vi "GetValuesFromRefs.vi"(11 "ChangeonFly":T2) -> (3 "output cluster":T1)   [LabVIEW 2023]
uses:
  TypeDefs/ChangeOnFly.ctl
  User_Vi/Settings.vi
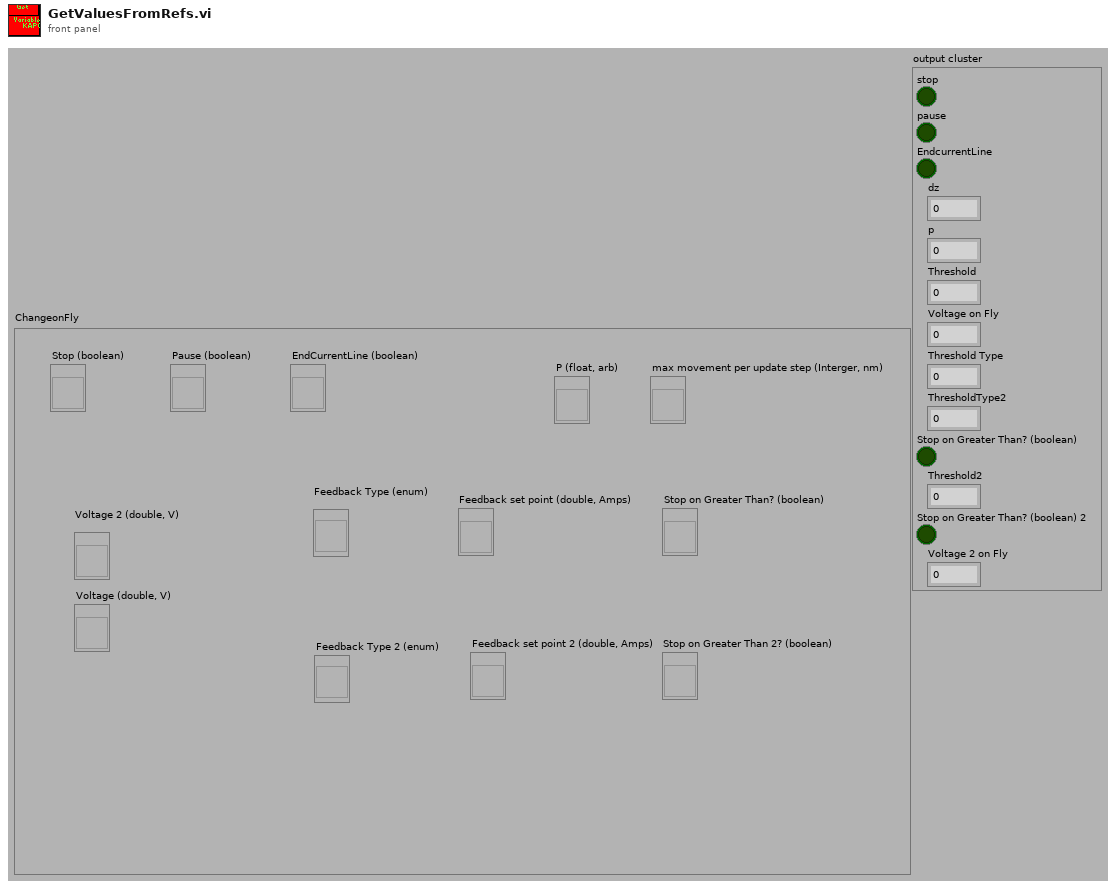
[diagram p1: front panel]
types:
  T1 = cluster{"stop":bool, "pause":bool, "EndcurrentLine":bool, "dz":i32, "p":fxp<+/-,32,1>, "Threshold":i64, "Voltage on Fly":i16, "Threshold Type":u8, "ThresholdType2":u8, "Stop on Greater Than? (boolean)":bool, "Threshold2":i64, "Stop on Greater Than? (boolean) 2":bool, "Voltage 2 on Fly":i16}
  T2 = typedef "ChangeOnFly.ctl" = cluster{"Stop (boolean)":refnum<vi>, "Pause (boolean)":refnum<vi>, "EndCurrentLine (boolean)":refnum<vi>, "max movement per update step (Interger, nm)":refnum<vi>, "P (float, arb)":refnum<vi>, "Feedback set point (double, Amps)":refnum<vi>, "Voltage (double, V)":refnum<vi>, "Feedback set point 2 (double, Amps)":refnum<vi>, "Stop on Greater Than 2? (boolean)":refnum<vi>, "Stop on Greater Than? (boolean)":refnum<vi>, "Voltage 2 (double, V)":refnum<vi>, "Feedback Type (enum)":refnum<vi>, "Feedback Type 2 (enum)":refnum<vi>}
  T3 = enum16{"AC Magnitude", "Current 1", "Current 2", "Phase"}
  T4 = typedef "Current Amplifier Settings.ctl" = dbl
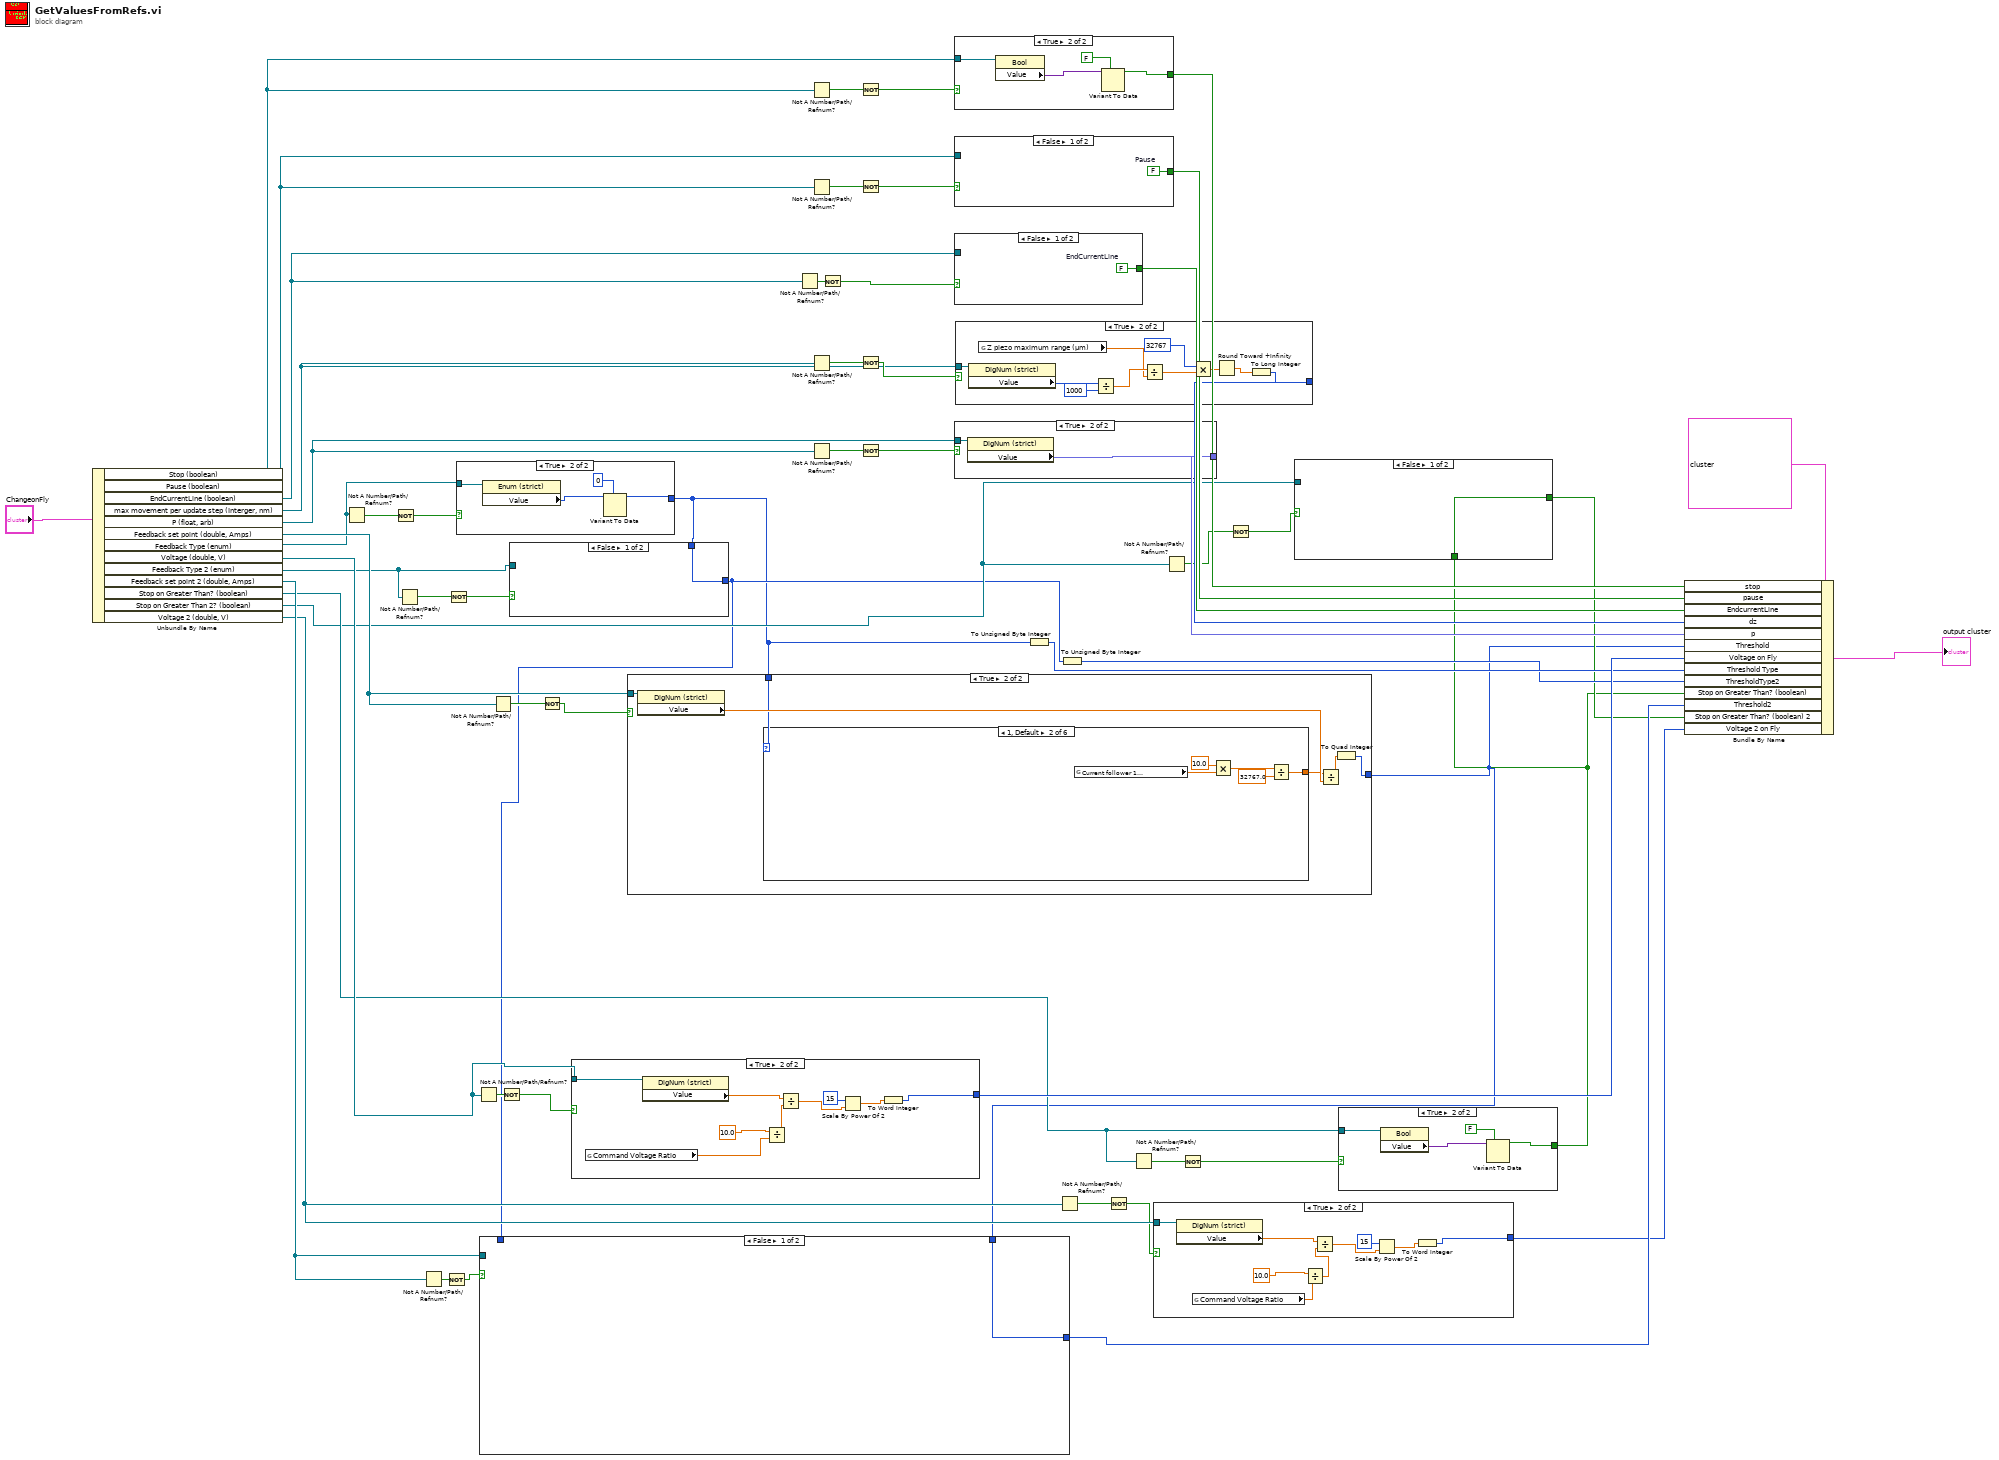
[diagram p0: block diagram]
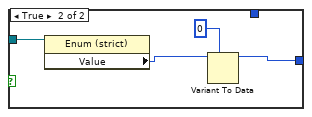
[diagram p2: hidden frame]
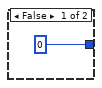
[diagram p3: hidden frame]
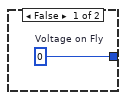
[diagram p4: hidden frame]
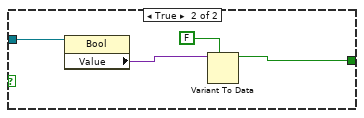
[diagram p5: hidden frame]
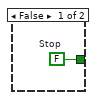
[diagram p6: hidden frame]
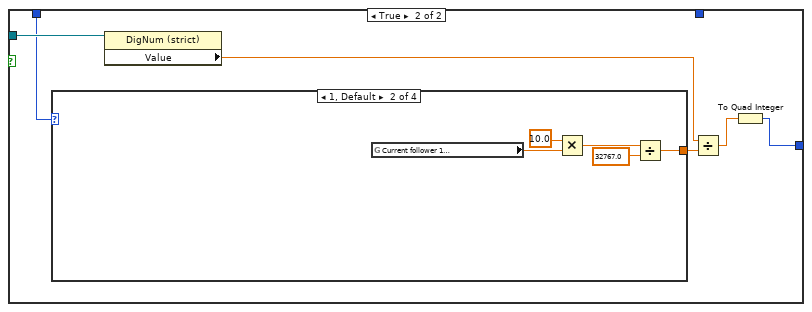
[diagram p7: hidden frame]
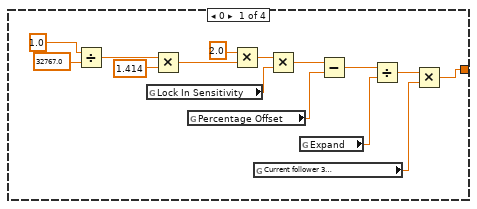
[diagram p8: hidden frame]
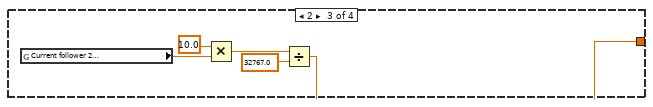
[diagram p9: hidden frame]
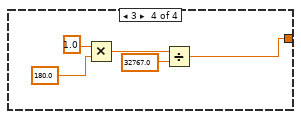
[diagram p10: hidden frame]
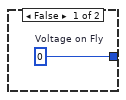
[diagram p11: hidden frame]
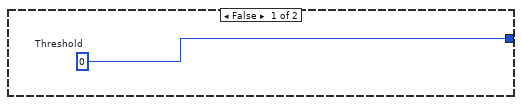
[diagram p12: hidden frame]
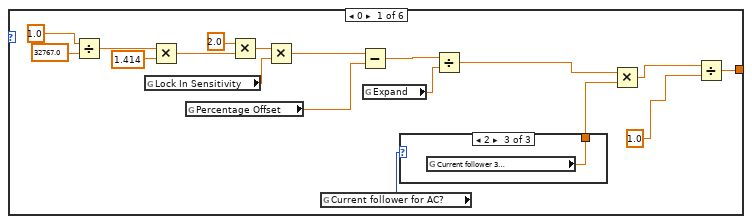
[diagram p13: hidden frame]
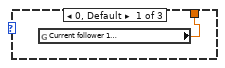
[diagram p14: hidden frame]
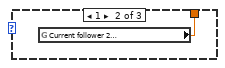
[diagram p15: hidden frame]
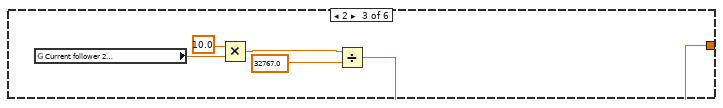
[diagram p16: hidden frame]
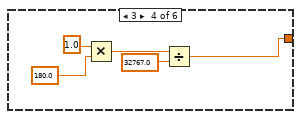
[diagram p17: hidden frame]
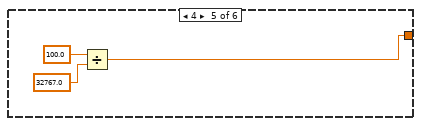
[diagram p18: hidden frame]
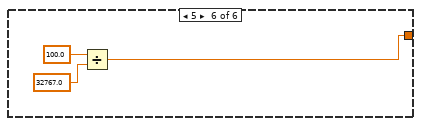
[diagram p19: hidden frame]
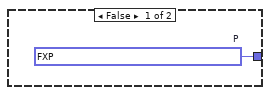
[diagram p20: hidden frame]
diagram:
  n1 = Unbundle By Name("ChangeonFly") -> ("Stop (boolean)"=w13:refnum<vi>, "Pause (boolean)"=w53:refnum<vi>, "EndCurrentLine (boolean)"=w50:refnum<vi>, "max movement per update step (Interger, nm)"=w47:refnum<vi>, "P (float, arb)"=w44:refnum<vi>, "Feedback set point (double, Amps)"=w36:refnum<vi>, "Feedback Type (enum)"=w10:refnum<vi>, "Voltage (double, V)"=w33:refnum<vi>, "Feedback Type 2 (enum)"=w9:refnum<vi>, "Feedback set point 2 (double, Amps)"=w25:refnum<vi>, "Stop on Greater Than? (boolean)"=w22:refnum<vi>, "Stop on Greater Than 2? (boolean)"=w19:refnum<vi>, "Voltage 2 (double, V)"=w15:refnum<vi>)
  n2 = Not A Number/Path/Refnum?(number/path/refnum=w10) -> (NaN/Path/Refnum?=w12:bool)
  n3 = Not(x=w12) -> (.not. x?=w11:bool)
  n4 = Not A Number/Path/Refnum?(number/path/refnum=w9) -> (NaN/Path/Refnum?=w8:bool)
  n5 = Not A Number/Path/Refnum?(number/path/refnum=w25) -> (NaN/Path/Refnum?=w30:bool)
  n6 = Not(x=w30) -> (.not. x?=w29:bool)
  n7 = Not(x=w8) -> (.not. x?=w7:bool)
  n8 = case shown="True" w11 {
    tunnel: w10 -> [_ w61]
    tunnel: [0 ("y") w59] -> w5
    frame False {
    }
    frame True {
      n9 = property on="Property Node" class="Enum (strict)"(reference=w61) -> ("Value"=w62:T3)  [unwired: 1 in, 2 out]
      n10 = Variant To Data(type=0 ("y"), Variant=w62) -> (data=w59:i32)  [unwired: 1 in, 1 out]
    }
  }
  n11 = Not A Number/Path/Refnum?(number/path/refnum=w33) -> (NaN/Path/Refnum?=w35:bool)
  n12 = Not A Number/Path/Refnum?(number/path/refnum=w36) -> (NaN/Path/Refnum?=w43:bool)
  n13 = Not(x=w35) -> (.not. x?=w34:bool)
  n14 = case shown="False" w7 {
    tunnel: [w63 w65] -> w6
    tunnel: w9 -> [_ w66]
    tunnel: w5 -> [w63 _]
    frame False {
    }
    frame True {
      n15 = property on="Property Node" class="Enum (strict)"(reference=w66) -> ("Value"=w67:T3)  [unwired: 1 in, 2 out]
      n16 = Variant To Data(type=0 ("y"), Variant=w67) -> (data=w65:i32)  [unwired: 1 in, 1 out]
    }
  }
  n17 = Not(x=w43) -> (.not. x?=w42:bool)
  n18 = case shown="True" w34 {
    tunnel: [w68 w72] -> w32
    tunnel: w33 -> [_ w77]
    frame False {
      w68 = i16 0  # Voltage on Fly
    }
    frame True {
      n19 = global read "Settings.vi" "Command Voltage Ratio"() -> (w69:dbl)
      n20 = property on="Property Node" class="DigNum (strict)"(reference=w77) -> ("Value"=w76:dbl)  [unwired: 1 in, 2 out]
      n21 = Divide(x=10.0 ("Max/Min Value [V]"), y=w69) -> (x/y=w70:dbl)
      n22 = Divide(x=w76, y=w70) -> (x/y=w74:dbl)
      n23 = Scale By Power Of 2(n=15, x=w74) -> (x*2^n=w73:dbl)
      n24 = To Word Integer(number=w73) -> (16bit integer=w72:i16)
    }
  }
  n25 = case shown="True" w42 {
    tunnel: w36 -> [_ w84]
    tunnel: [w78 w79] -> w4
    tunnel: w5 -> [_ w81]
    frame False {
      w78 = i64 0  # Threshold
    }
    frame True {
      n26 = property on="Property Node" class="DigNum (strict)"(reference=w84) -> ("Value"=w82:dbl)  [unwired: 1 in, 2 out]
      n27 = case shown="1, Default" w81 {
        tunnel: [w88 w108 w111 w116 w121 w124] -> w83
        frame 0 {
          n28 = Divide(x=1.0, y=32767.0 ("n")) -> (x/y=w94:dbl)
          n29 = global read "Settings.vi" "Lock In Sensitivity"() -> (w101:dbl)
          n30 = Multiply(x=w94, y=1.414) -> (x*y=w95:dbl)
          n31 = global read "Settings.vi" "Percentage Offset"() -> (w91:dbl)
          n32 = Multiply(x=2.0 ("y"), y=w95) -> (x*y=w100:dbl)
          n33 = Multiply(x=w100, y=w101) -> (x*y=w102:dbl)
          n34 = global read "Settings.vi" "Current follower for AC?"() -> (w85:u8)
          n35 = Subtract(x=w102, y=w91) -> (x-y=w97:dbl)
          n36 = global read "Settings.vi" "Expand"() -> (w98:dbl)
          n37 = case shown="2" w85 {
            tunnel: [w103 w104 w105] -> w89
            frame 0, Default {
              n38 = global read "Settings.vi" "Current follower 1\n (AI-3)"() -> (w103:T4)
            }
            frame 1 {
              n39 = global read "Settings.vi" "Current follower 2 \n(AI-4)"() -> (w104:T4)
            }
            frame 2 {
              n40 = global read "Settings.vi" "Current follower 3\n(AI-6)"() -> (w105:T4)
            }
          }
          n41 = Divide(x=w97, y=w98) -> (x/y=w99:dbl)
          n42 = Multiply(x=w99, y=w89) -> (x*y=w87:T4)
          n43 = Divide(x=w87, y=1.0 ("x")) -> (x/y=w88:T4)
        }
        frame 1, Default {
          n44 = global read "Settings.vi" "Current follower 1\n (AI-3)"() -> (w110:T4)
          n45 = Multiply(x=10.0 ("Max Value [um]"), y=w110) -> (x*y=w107:T4)
          n46 = Divide(x=w107, y=32767.0 ("n")) -> (x/y=w108:T4)
        }
        frame 2 {
          n47 = global read "Settings.vi" "Current follower 2 \n(AI-4)"() -> (w115:T4)
          n48 = Multiply(x=10.0 ("Max Value [um]"), y=w115) -> (x*y=w113:T4)
          n49 = Divide(x=w113, y=32767.0 ("n")) -> (x/y=w111:T4)
        }
        frame 3 {
          n50 = Multiply(x=1.0 ("Max Value [um]"), y=180.0 ("Max Value [um]")) -> (x*y=w119:dbl)
          n51 = Divide(x=w119, y=32767.0 ("n")) -> (x/y=w116:dbl)
        }
        frame 4 {
          n52 = Divide(x=100.0, y=32767.0 ("x")) -> (x/y=w121:dbl)
        }
        frame 5 {
          n53 = Divide(x=100.0, y=32767.0 ("x")) -> (x/y=w124:dbl)
        }
      }
      n54 = Divide(x=w82, y=w83) -> (x/y=w80:T4)
      n55 = To Quad Integer(1:w80) -> (0:w79:i64)
    }
  }
  n56 = case shown="False" w29 {
    tunnel: [w127 w128] -> w26
    tunnel: w25 -> [_ w131]
    tunnel: w6 -> [_ w130]
    tunnel: w4 -> [w127 _]
    frame False {
    }
    frame True {
      n57 = case shown="1, Default" w130 {
        tunnel: [w134 w151 w154 w159] -> w133
        frame 0 {
          n58 = Divide(x=1.0, y=32767.0 ("n")) -> (x/y=w140:dbl)
          n59 = global read "Settings.vi" "Lock In Sensitivity"() -> (w147:dbl)
          n60 = Multiply(x=w140, y=1.414) -> (x*y=w141:dbl)
          n61 = global read "Settings.vi" "Percentage Offset"() -> (w136:dbl)
          n62 = Multiply(x=2.0 ("y"), y=w141) -> (x*y=w146:dbl)
          n63 = global read "Settings.vi" "Current follower 3\n(AI-6)"() -> (w138:T4)
          n64 = Multiply(x=w146, y=w147) -> (x*y=w148:dbl)
          n65 = global read "Settings.vi" "Expand"() -> (w144:dbl)
          n66 = Subtract(x=w148, y=w136) -> (x-y=w143:dbl)
          n67 = Divide(x=w143, y=w144) -> (x/y=w145:dbl)
          n68 = Multiply(x=w145, y=w138) -> (x*y=w134:T4)
        }
        frame 1, Default {
          n69 = global read "Settings.vi" "Current follower 1\n (AI-3)"() -> (w153:T4)
          n70 = Multiply(x=10.0 ("Max Value [um]"), y=w153) -> (x*y=w150:T4)
          n71 = Divide(x=w150, y=32767.0 ("n")) -> (x/y=w151:T4)
        }
        frame 2 {
          n72 = global read "Settings.vi" "Current follower 2 \n(AI-4)"() -> (w158:T4)
          n73 = Multiply(x=10.0 ("Max Value [um]"), y=w158) -> (x*y=w156:T4)
          n74 = Divide(x=w156, y=32767.0 ("n")) -> (x/y=w154:T4)
        }
        frame 3 {
          n75 = Multiply(x=1.0 ("Max Value [um]"), y=180.0 ("Max Value [um]")) -> (x*y=w162:dbl)
          n76 = Divide(x=w162, y=32767.0 ("n")) -> (x/y=w159:dbl)
        }
      }
      n77 = property on="Property Node" class="DigNum (strict)"(reference=w131) -> ("Value"=w132:dbl)  [unwired: 1 in, 2 out]
      n78 = Divide(x=w132, y=w133) -> (x/y=w129:T4)
      n79 = To Quad Integer(1:w129) -> (0:w128:i64)
    }
  }
  n80 = Not A Number/Path/Refnum?(number/path/refnum=w50) -> (NaN/Path/Refnum?=w52:bool)
  n81 = Not A Number/Path/Refnum?(number/path/refnum=w13) -> (NaN/Path/Refnum?=w57:bool)
  n82 = Not A Number/Path/Refnum?(number/path/refnum=w53) -> (NaN/Path/Refnum?=w54:bool)
  n83 = Not A Number/Path/Refnum?(number/path/refnum=w47) -> (NaN/Path/Refnum?=w48:bool)
  n84 = Not A Number/Path/Refnum?(number/path/refnum=w44) -> (NaN/Path/Refnum?=w46:bool)
  n85 = Not(x=w52) -> (.not. x?=w51:bool)
  n86 = Not(x=w57) -> (.not. x?=w56:bool)
  n87 = Not(x=w54) -> (.not. x?=w55:bool)
  n88 = Not(x=w48) -> (.not. x?=w49:bool)
  n89 = Not(x=w46) -> (.not. x?=w45:bool)
  n90 = case shown="True" w56 {
    tunnel: [w164 w165] -> w41
    tunnel: w13 -> [_ w166]
    frame False {
      w164 = FALSE  # Stop
    }
    frame True {
      n91 = property on="Property Node" class="Bool"(reference=w166) -> ("Value"=w168:variant)  [unwired: 1 in, 2 out]
      n92 = Variant To Data(type=FALSE ("stop"), Variant=w168) -> (data=w165:bool)  [unwired: 1 in, 1 out]
    }
  }
  n93 = case shown="False" w55 {
    tunnel: [w169 w170] -> w40
    tunnel: w53 -> [_ w171]
    frame False {
      w169 = FALSE  # Pause
    }
    frame True {
      n94 = property on="Property Node" class="Bool"(reference=w171) -> ("Value"=w173:variant)  [unwired: 1 in, 2 out]
      n95 = Variant To Data(type=FALSE ("stop"), Variant=w173) -> (data=w170:bool)  [unwired: 1 in, 1 out]
    }
  }
  n96 = case shown="False" w51 {
    tunnel: [w174 w175] -> w39
    tunnel: w50 -> [_ w176]
    frame False {
      w174 = FALSE  # EndCurrentLine
    }
    frame True {
      n97 = property on="Property Node" class="Bool"(reference=w176) -> ("Value"=w178:variant)  [unwired: 1 in, 2 out]
      n98 = Variant To Data(type=FALSE ("stop"), Variant=w178) -> (data=w175:bool)  [unwired: 1 in, 1 out]
    }
  }
  n99 = case shown="True" w45 {
    tunnel: w44 -> [_ w181]
    tunnel: [w179 w180] -> w37
    frame False {
      w179 = fxp<+/-,32,1> 0.0  # P
    }
    frame True {
      n100 = property on="Property Node" class="DigNum (strict)"(reference=w181) -> ("Value"=w180:fxp<+/-,32,1>)  [unwired: 1 in, 2 out]
    }
  }
  n101 = case shown="True" w49 {
    tunnel: w47 -> [_ w192]
    tunnel: [w182 w183] -> w38
    frame False {
      w182 = 0  # UpperdZ
    }
    frame True {
      n102 = property on="Property Node" class="DigNum (strict)"(reference=w192) -> ("Value"=w191:i32)  [unwired: 1 in, 2 out]
      n103 = global read "Settings.vi" "Z piezo maximum range (µm)"() -> (w188:dbl)
      n104 = Divide(x=w191, y=1000) -> (x/y=w189:dbl)
      n105 = Divide(x=w189, y=w188) -> (x/y=w187:dbl)
      n106 = Multiply(x=i16 32767, y=w187) -> (x*y=w185:dbl)
      n107 = Round Toward +Infinity(x=w185) -> (ceil(x): smallest int >= x=w184:dbl)
      n108 = To Long Integer(number=w184) -> (32bit integer=w183:i32)
    }
  }
  n109 = To Unsigned Byte Integer(number=w5) -> (unsigned 8bit integer=w28:u8)
  n110 = Not A Number/Path/Refnum?(number/path/refnum=w15) -> (NaN/Path/Refnum?=w16:bool)
  n111 = To Unsigned Byte Integer(number=w6) -> (unsigned 8bit integer=w27:u8)
  n112 = Not(x=w16) -> (.not. x?=w14:bool)
  n113 = Not A Number/Path/Refnum?(number/path/refnum=w22) -> (NaN/Path/Refnum?=w23:bool)
  n114 = case shown="True" w14 {
    tunnel: [w193 w197] -> w17
    tunnel: w15 -> [_ w202]
    frame False {
      w193 = i16 0  # Voltage on Fly
    }
    frame True {
      n115 = property on="Property Node" class="DigNum (strict)"(reference=w202) -> ("Value"=w201:dbl)  [unwired: 1 in, 2 out]
      n116 = global read "Settings.vi" "Command Voltage Ratio"() -> (w196:dbl)
      n117 = Divide(x=10.0 ("Max/Min Value [V]"), y=w196) -> (x/y=w194:dbl)
      n118 = Divide(x=w201, y=w194) -> (x/y=w199:dbl)
      n119 = Scale By Power Of 2(n=15, x=w199) -> (x*2^n=w198:dbl)
      n120 = To Word Integer(number=w198) -> (16bit integer=w197:i16)
    }
  }
  n121 = Not A Number/Path/Refnum?(number/path/refnum=w19) -> (NaN/Path/Refnum?=w21:bool)
  n122 = Not(x=w23) -> (.not. x?=w24:bool)
  n123 = Not(x=w21) -> (.not. x?=w20:bool)
  n124 = case shown="True" w24 {
    tunnel: [w203 w204] -> w3
    tunnel: w22 -> [_ w205]
    frame False {
      w203 = FALSE  # Stop
    }
    frame True {
      n125 = property on="Property Node" class="Bool"(reference=w205) -> ("Value"=w207:variant)  [unwired: 1 in, 2 out]
      n126 = Variant To Data(type=FALSE ("stop"), Variant=w207) -> (data=w204:bool)  [unwired: 1 in, 1 out]
    }
  }
  n127 = case shown="False" w20 {
    tunnel: [w208 w209] -> w18
    tunnel: w19 -> [_ w210]
    tunnel: w3 -> [w208 _]
    frame False {
    }
    frame True {
      n128 = property on="Property Node" class="Bool"(reference=w210) -> ("Value"=w212:variant)  [unwired: 1 in, 2 out]
      n129 = Variant To Data(type=FALSE ("stop"), Variant=w212) -> (data=w209:bool)  [unwired: 1 in, 1 out]
    }
  }
  n130 = Bundle By Name(cluster=T1 {"stop"=FALSE, "pause"=FALSE, "EndcurrentLine"=FALSE, "dz"=0, "p"=0.0, "Threshold"=0, "Voltage on Fly"=0, "Threshold Type"=0, "ThresholdType2"=0, "Stop on Greater Than? (boolean)"=FALSE, "Threshold2"=0, "Stop on Greater Than? (boolean) 2"=FALSE, "Voltage 2 on Fly"=0} ("input cluster"), "stop"=w41, "pause"=w40, "EndcurrentLine"=w39, "dz"=w38, "p"=w37, "Threshold"=w4, "Voltage on Fly"=w32, "Threshold Type"=w28, "ThresholdType2"=w27, "Stop on Greater Than? (boolean)"=w3, "Threshold2"=w26, "Stop on Greater Than? (boolean) 2"=w18, "Voltage 2 on Fly"=w17) -> (→"output cluster":T1)
